vi "Test Operations.vi"(11 "Error in":errorcluster) -> (15 "Error out":errorcluster)   [LabVIEW 2020, in "LogicalComparisonTest.lvlib"]
doc: "This VI is the validating VI for the Logical comparison"
uses:
  LogicalComparisonTest.lvlib
  <vilib>/SLL Drona/APIs/Stimulus/ControlValue/SetValueAuto.vi
  <vilib>/SLL Drona/APIs/Assert/AssertControlValue/Equal.vi
  <vilib>/SLL Drona/APIs/Stimulus/VI/CloseVI.vi
  <vilib>/Utility/error.llb/Error Cluster From Error Code.vi
  <vilib>/ErrorRing/Error Ring.xnode
  <vilib>/SLL Drona/Drona.lvlib
  <vilib>/addons/_JKI Toolkits/Caraya/classes/Test/Test.lvclass
  <vilib>/SLL Drona/APIs/Stimulus/ControlValue/ControlValue.lvlib
  <vilib>/SLL Drona/APIs/Assert/AssertControlValue/AssertControlValue.lvlib
  <vilib>/Wiresmith Technology/G CLI/CLI Class/CLI.lvclass
  <vilib>/SLL Drona/APIs/Stimulus/VI/VI.lvlib
panel:
  # "LOGICAL COMPARISION TEST"
  # "Testing........."
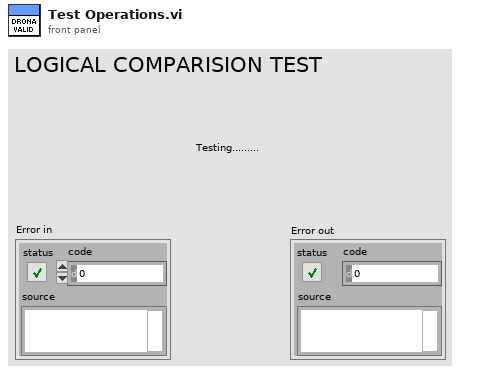
[diagram p1: front panel]
types:
  T1 = cluster{"A":dbl, "B":dbl, "Operations":enum16{"A>B", "A<B", "A>=B", "A<=B", "A=B", "A!=B"}, "Result":bool}[]
  T2 = enum16{"A>B", "A<B", "A>=B", "A<=B", "A=B", "A!=B"}
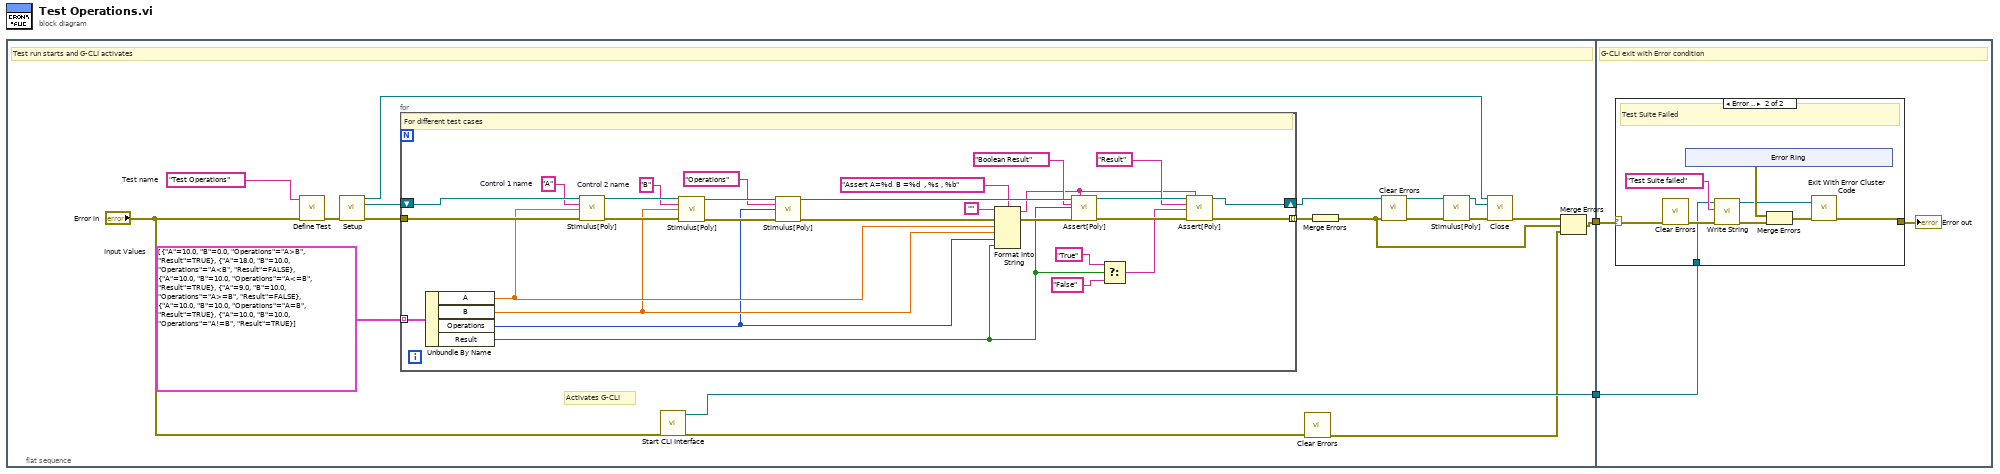
[diagram p0: block diagram]
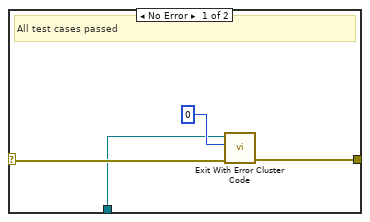
[diagram p2: hidden frame]
diagram:
  n1 = flat-sequence {
    tunnel: [w11] -> w2
    tunnel: [w9] -> w1
    tunnel: w2 -> [w52]
    tunnel: w1 -> [w50]
    frame #0 {
      w8 = "Test Operations"  # Test name
      w17 = T1 [{"A"=10.0, "B"=0.0, "Operations"=enum."A>B", "Result"=TRUE}, {"A"=18.0, "B"=10.0, "Operations"=enum."A<B", "Result"=FALSE}, {"A"=10.0, "B"=10.0, "Operations"=enum."A<=B", "Result"=TRUE}, {"A"=9.0, "B"=10.0, "Operations"=enum."A>=B", "Result"=FALSE}, {"A"=10.0, "B"=10.0, "Operations"=enum."A=B", "Result"=TRUE}, {"A"=10.0, "B"=10.0, "Operations"=enum."A!=B", "Result"=TRUE}]  # Input Values
      # "Activates G-CLI"
      # "Test run starts and G-CLI activates"
      n2 = call <vilib>:"Define Test.vi"("error in (no error)"="Error in", "Label (VI Title)"=w8) -> ("error out"=w20:errorcluster)  [unwired: 8 in, 1 out]
      n3 = call <vilib>:"Setup.vi"("error in"=w20) -> ("Application Ref"=w16:refnum<vi>, "VI Reference Out"=w18:refnum<vi>, "error out"=w19:errorcluster)  [unwired: 12 in]
      n4 = for {
        shift-right: [w33] -> w15
        shift-left: w18 -> [w46]
        tunnel: w17 -> [w43] mode=indexing
        tunnel: w19 -> [w49]
        tunnel: [w21] -> w12 mode=indexing
        w40 = "B"  # Control 2 name
        w42 = "A"  # Control 1 name
        # "For different test cases"
        n5 = Unbundle By Name(w43) -> ("A"=w25:dbl, "B"=w24:dbl, "Operations"=w23:T2, "Result"=w22:bool)
        n6 = call-poly <vilib>:"Stimulus[Poly].vi"("VI Reference In"=w46, "Control Path"=w42, "Value (Signaling)"=w25, "error in"=w49) -> ("VI Reference Out"=w41:refnum<vi>, "error out"=w48:errorcluster)  [unwired: 10 in]
        n7 = call-poly <vilib>:"Stimulus[Poly].vi"("VI Reference In"=w41, "Control Path"=w40, "Value (Signaling)"=w24, "error in"=w48) -> ("VI Reference Out"=w39:refnum<vi>, "error out"=w47:errorcluster)  [unwired: 10 in]
        n8 = call-poly <vilib>:"Stimulus[Poly].vi"("VI Reference In"=w39, "Control Path"="Operations", "Value (Signaling)"=w23, "error in"=w47) -> ("VI Reference Out"=w37:refnum<vi>, "error out"=w45:errorcluster)  [unwired: 10 in]
        n9 = Format Into String(format string="Assert A=%d  B =%d  , %s , %b", initial string="", error in=w45, w25, w24, w23, w22) -> (resulting string=w31:string, error out=w44:errorcluster)
        n10 = call-poly <vilib>:"Assert[Poly].vi"("VI Reference In"=w37, "Test Label"=w31, "Control Path"="Boolean Result", "Control Value"=w22, "Error In"=w44) -> ("VI Reference Out"=w34:refnum<vi>, "Error Out"=w35:errorcluster)  [unwired: 9 in]
        n11 = Select(t="True", s=w22, f="False") -> (s? t:f=w26:string)
        n12 = call-poly <vilib>:"Assert[Poly].vi"("VI Reference In"=w34, "Test Label"=w31, "Control Path"="Result", "Control Value"=w26, "Error In"=w35) -> ("VI Reference Out"=w33:refnum<vi>, "Error Out"=w21:errorcluster)  [unwired: 9 in]
      }
      n13 = call <vilib>:"Start CLI Interface.vi"("error in (no error)"="Error in") -> ("error out"=w10:errorcluster, "CLI out"=w9:refnum<class "CLI.lvclass">)  [unwired: 7 in, 2 out]
      n14 = call <vilib>:"Clear Errors.vi"("error in (no error)"=w10) -> ("error out"=w5:errorcluster)  [unwired: 5 in, 1 out]
      n15 = Merge Errors(w12) -> (w6:errorcluster)
      n16 = call <vilib>:"Clear Errors.vi"("error in (no error)"=w6) -> ("error out"=w7:errorcluster)  [unwired: 5 in, 1 out]
      n17 = call-poly <vilib>:"Stimulus[Poly].vi"("VI Reference In"=w15, "error in"=w7) -> ("VI Reference Out"=w13:refnum<vi>, "error out"=w14:errorcluster)  [unwired: 12 in]
      n18 = call <vilib>:"Close.vi"("Application Ref"=w16, "VI Reference"=w13, "error in"=w14) -> ("error out"=w3:errorcluster)  [unwired: 12 in]
      n19 = Merge Errors(w3, w6, w5) -> (w11:errorcluster)
    }
    frame #1 {
      # "G-CLI exit with Error condition"
      n20 = case shown="Error .." w52 {
        selector: w52 -> [w56 w63]
        tunnel: w50 -> [w54 w58]
        tunnel: [w53 w65] -> w51
        frame No Error {
          # "All test cases passed"
          n21 = call <vilib>:"Exit With Error Cluster Code.vi"("error in (no error)"=w56, "No Error Code (0)"=0, "CLI in"=w54) -> ("error out"=w53:errorcluster)  [unwired: 8 in]
        }
        frame Error {
          # "Test Suite Failed"
          n22 = call <vilib>:"Clear Errors.vi"("error in (no error)"=w63) -> ("error out"=w62:errorcluster)  [unwired: 5 in, 1 out]
          n23 = xnode "Error Ring"() -> ("error out"=w61:errorcluster)
          n24 = call <vilib>:"Write String.vi"("error in (no error)"=w62, "Text to Write"="Test Suite failed", "CLI in"=w58) -> ("error out"=w60:errorcluster, "CLI out"=w57:refnum<class "CLI.lvclass">)  [unwired: 7 in]
          n25 = Merge Errors(w61, w60) -> (w59:errorcluster)
          n26 = call <vilib>:"Exit With Error Cluster Code.vi"("error in (no error)"=w59, "CLI in"=w57) -> ("error out"=w65:errorcluster)  [unwired: 9 in]
        }
      }
      "Error out" <- w51
    }
  }
